vi "WebView2 Viewer.vi"(2 "ProjectRef":refnum<vi>, 4 "Extra Scripts":string, 5 "FileDependency In":map{path, T1}(c390), 6 "Options":string, 7 "OpenWebBrowser(False)":bool, 8 "error in":errorcluster, 9 "Embedd VISJS Librarya in HTMl File(False)":bool, 10 "HTMLFilePath":path, 11 "LibraryDependency":map{path, T3}(c390)) -> (0 "error out":errorcluster, 3 "HTMLFileContent":string)   [LabVIEW 2020, in "WebView2-Viewer.lvlib"] (continued)
if(this.selected=g,void 0!==this.imageObjAlt&&t){var A=this.imageObj;this.imageObj=this.imageObjAlt,this.imageObjAlt=A}}},{key:\"_getImagePadding\",value:function(){var g={top:0,right:0,bottom:0,left:0};if(this.options.imagePadding){var t=this.options.imagePadding;\"object\"==yd(t)?(g.top=t.top,g.right=t.right,g.bottom=t.bottom,g.left=t.left):(g.top=t,g.right=t,g.bottom=t,g.left=t)}return g}},{key:\"_resizeImage\",value:function(){var g,t;if(!1===this.options.shapeProperties.useImageSize){var A=1,e=1;this.imageObj.width&&this.imageObj.height&&(this.imageObj.width>this.imageObj.height?A=this.imageObj.width/this.imageObj.height:e=this.imageObj.height/this.imageObj.width),g=2*this.options.size*A,t=2*this.options.size*e}else{var C=this._getImagePadding();g=this.imageObj.width+C.left+C.right,t=this.imageObj.height+C.top+C.bottom}this.width=g,this.height=t,this.radius=.5*this.width}},{key:\"_drawRawCircle\",value:function(g,t,A,e){this.initContextForDraw(g,e),Le(g,t,A,e.size),this.performFill(g,e)}},{key:\"_drawImageAtPosition\",value:function(g,t){if(0!=this.imageObj.width){g.globalAlpha=void 0!==t.opacity?t.opacity:1,this.enableShadow(g,t);var A=1;!0===this.options.shapeProperties.interpolation&&(A=this.imageObj.width/this.width/this.body.view.scale);var e=this._getImagePadding(),C=this.left+e.left,I=this.top+e.top,i=this.width-e.left-e.right,o=this.height-e.top-e.bottom;this.imageObj.drawImageAtPosition(g,A,C,I,i,o),this.disableShadow(g,t)}}},{key:\"_drawImageLabel\",value:function(g,t,A,e,C){var I=0;if(void 0!==this.height){I=.5*this.height;var i=this.labelModule.getTextSize(g,e,C);i.lineCount>=1&&(I+=i.height/2)}var o=A+I;this.options.label&&(this.labelOffset=I),this.labelModule.draw(g,t,o,e,C,\"hanging\")}}]),A}($D);function CN(g){var t=function(){if(\"undefined\"==typeof Reflect||!MT)return!1;if(MT.sham)return!1;if(\"function\"==typeof Proxy)return!0;try{return Boolean.prototype.valueOf.call(MT(Boolean,[],(function(){}))),!0}catch(g){return!1}}();return function(){var A,e=nb(g);if(t){var C=nb(this).constructor;A=MT(e,arguments,C)}else A=e.apply(this,arguments);return Ib(this,A)}}var IN=function(g){Cb(A,g);var t=CN(A);function A(g,e,C){var I;return cn(this,A),(I=t.call(this,g,e,C))._setMargins(C),I}return kd(A,[{key:\"resize\",value:function(g){var t=arguments.length>1&&void 0!==arguments[1]?arguments[1]:this.selected,A=arguments.length>2&&void 0!==arguments[2]?arguments[2]:this.hover;if(this.needsRefresh(t,A)){var e=this.getDimensionsFromLabel(g,t,A),C=Math.max(e.width+this.margin.right+this.margin.left,e.height+this.margin.top+this.margin.bottom);this.options.size=C/2,this.width=C,this.height=C,this.radius=this.width/2}}},{key:\"draw\",value:function(g,t,A,e,C,I){this.resize(g,e,C),this.left=t-this.width/2,this.top=A-this.height/2,this._drawRawCircle(g,t,A,I),this.updateBoundingBox(t,A),this.labelModule.draw(g,this.left+this.textSize.width/2+this.margin.left,A,e,C)}},{key:\"updateBoundingBox\",value:function(g,t){this.boundingBox.top=t-this.options.size,this.boundingBox.left=g-this.options.size,this.boundingBox.right=g+this.options.size,this.boundingBox.bottom=t+this.options.size}},{key:\"distanceToBorder\",value:function(g){return g&&this.resize(g),.5*this.width}}]),A}(eN);function iN(g){var t=function(){if(\"undefined\"==typeof Reflect||!MT)return!1;if(MT.sham)return!1;if(\"function\"==typeof Proxy)return!0;try{return Boolean.prototype.valueOf.call(MT(Boolean,[],(function(){}))),!0}catch(g){return!1}}();return function(){var A,e=nb(g);if(t){var C=nb(this).constructor;A=MT(e,arguments,C)}else A=e.apply(this,arguments);return Ib(this,A)}}var oN=function(g){Cb(A,g);var t=iN(A);function A(g,e,C,I,i){var o;return cn(this,A),(o=t.call(this,g,e,C)).setImages(I,i),o}return kd(A,[{key:\"resize\",value:function(g){var t=arguments.length>1&&void 0!==arguments[1]?arguments[1]:this.selected,A=arguments.length>2&&void 0!==arguments[2]?arguments[2]:this.hover;if(void 0===this.imageObj.src||void 0===this.imageObj.width||void 0===this.imageObj.height){var e=2*this.options.size;return this.width=e,this.height=e,void(this.radius=.5*this.width)}this.needsRefresh(t,A)&&this._resizeImage()}},{key:\"draw\",value:function(g,t,A,e,C,I){this.switchImages(e),this.resize();var i=t,o=A;\"top-left\"===this.options.shapeProperties.coordinateOrigin?(this.left=t,this.top=A,i+=this.width/2,o+=this.height/2):(this.left=t-this.width/2,this.top=A-this.height/2),this._drawRawCircle(g,i,o,I),g.save(),g.clip(),this._drawImageAtPosition(g,I),g.restore(),this._drawImageLabel(g,i,o,e,C),this.updateBoundingBox(t,A)}},{key:\"updateBoundingBox\",value:function(g,t){\"top-left\"===this.options.shapeProperties.coordinateOrigin?(this.boundingBox.top=t,this.boundingBox.left=g,this.boundingBox.right=g+2*this.options.size,this.boundingBox.bottom=t+2*this.options.size):(this.boundingBox.top=t-this.options.size,this.boundingBox.left=g-this.options.size,this.boundingBox.right=g+this.options.size,this.boundingBox.bottom=t+this.options.size),this.boundingBox.left=Math.min(this.boundingBox.left,this.labelModule.size.left),this.boundingBox.right=Math.max(this.boundingBox.right,this.labelModule.size.left+this.labelModule.size.width),this.boundingBox.bottom=Math.max(this.boundingBox.bottom,this.boundingBox.bottom+this.labelOffset)}},{key:\"distanceToBorder\",value:function(g){return g&&this.resize(g),.5*this.width}}]),A}(eN);function nN(g){var t=function(){if(\"undefined\"==typeof Reflect||!MT)return!1;if(MT.sham)return!1;if(\"function\"==typeof Proxy)return!0;try{return Boolean.prototype.valueOf.call(MT(Boolean,[],(function(){}))),!0}catch(g){return!1}}();return function(){var A,e=nb(g);if(t){var C=nb(this).constructor;A=MT(e,arguments,C)}else A=e.apply(this,arguments);return Ib(this,A)}}var rN=function(g){Cb(A,g);var t=nN(A);function A(g,e,C){return cn(this,A),t.call(this,g,e,C)}return kd(A,[{key:\"resize\",value:function(g){var t=arguments.length>1&&void 0!==arguments[1]?arguments[1]:this.selected,A=arguments.length>2&&void 0!==arguments[2]?arguments[2]:this.hover,e=arguments.length>3&&void 0!==arguments[3]?arguments[3]:{size:this.options.size};if(this.needsRefresh(t,A)){var C,I;this.labelModule.getTextSize(g,t,A);var i=2*e.size;this.width=null!==(C=this.customSizeWidth)&&void 0!==C?C:i,this.height=null!==(I=this.customSizeHeight)&&void 0!==I?I:i,this.radius=.5*this.width}}},{key:\"_drawShape\",value:function(g,t,A,e,C,I,i,o){var n,r=this;return this.resize(g,I,i,o),this.left=e-this.width/2,this.top=C-this.height/2,this.initContextForDraw(g,o),(n=t,Object.prototype.hasOwnProperty.call(Ue,n)?Ue[n]:function(g){for(var t=arguments.length,A=new Array(t>1?t-1:0),e=1;e<t;e++)A[e-1]=arguments[e];CanvasRenderingContext2D.prototype[n].call(g,A)})(g,e,C,o.size),this.performFill(g,o),void 0!==this.options.icon&&void 0!==this.options.icon.code&&(g.font=(I?\"bold \":\"\")+this.height/2+\"px \"+(this.options.icon.face||\"FontAwesome\"),g.fillStyle=this.options.icon.color||\"black\",g.textAlign=\"center\",g.textBaseline=\"middle\",g.fillText(this.options.icon.code,e,C)),{drawExternalLabel:function(){if(void 0!==r.options.label){r.labelModule.calculateLabelSize(g,I,i,e,C,\"hanging\");var t=C+.5*r.height+.5*r.labelModule.size.height;r.labelModule.draw(g,e,t,I,i,\"hanging\")}r.updateBoundingBox(e,C)}}}},{key:\"updateBoundingBox\",value:function(g,t){this.boundingBox.top=t-this.options.size,this.boundingBox.left=g-this.options.size,this.boundingBox.right=g+this.options.size,this.boundingBox.bottom=t+this.options.size,void 0!==this.options.label&&this.labelModule.size.width>0&&(this.boundingBox.left=Math.min(this.boundingBox.left,this.labelModule.size.left),this.boundingBox.right=Math.max(this.boundingBox.right,this.labelModule.size.left+this.labelModule.size.width),this.boundingBox.bottom=Math.max(this.boundingBox.bottom,this.boundingBox.bottom+this.labelModule.size.height))}}]),A}($D);function sN(g,t){var A=Lh(g);if(BT){var e=BT(g);t&&(e=pc(e).call(e,(function(t){return WT(g,t).enumerable}))),A.push.apply(A,e)}return A}function aN(g){for(var t=1;t<arguments.length;t++){var A,e,C=null!=arguments[t]?arguments[t]:{};t%2?Cl(A=sN(Object(C),!0)).call(A,(function(t){rb(g,t,C[t])})):HT?AD(g,HT(C)):Cl(e=sN(Object(C))).call(e,(function(t){fT(g,t,WT(C,t))}))}return g}function dN(g){var t=function(){if(\"undefined\"==typeof Reflect||!MT)return!1;if(MT.sham)return!1;if(\"function\"==typeof Proxy)return!0;try{return Boolean.prototype.valueOf.call(MT(Boolean,[],(function(){}))),!0}catch(g){return!1}}();return function(){var A,e=nb(g);if(t){var C=nb(this).constructor;A=MT(e,arguments,C)}else A=e.apply(this,arguments);return Ib(this,A)}}var hN=function(g){Cb(A,g);var t=dN(A);function A(g,e,C,I){var i;return cn(this,A),(i=t.call(this,g,e,C,I)).ctxRenderer=I,i}return kd(A,[{key:\"draw\",value:function(g,t,A,e,C,I){this.resize(g,e,C,I),this.left=t-this.width/2,this.top=A-this.height/2,g.save();var i=this.ctxRenderer({ctx:g,id:this.options.id,x:t,y:A,state:{selected:e,hover:C},style:aN({},I),label:this.options.label});if(null!=i.drawNode&&i.drawNode(),g.restore(),i.drawExternalLabel){var o=i.drawExternalLabel;i.drawExternalLabel=function(){g.save(),o(),g.restore()}}return i.nodeDimensions&&(this.customSizeWidth=i.nodeDimensions.width,this.customSizeHeight=i.nodeDimensions.height),i}},{key:\"distanceToBorder\",value:function(g,t){return this._distanceToBorder(g,t)}}]),A}(rN);function lN(g){var t=function(){if(\"undefined\"==typeof Reflect||!MT)return!1;if(MT.sham)return!1;if(\"function\"==typeof Proxy)return!0;try{return Boolean.prototype.valueOf.call(MT(Boolean,[],(function(){}))),!0}catch(g){return!1}}();return function(){var A,e=nb(g);if(t){var C=nb(this).constructor;A=MT(e,arguments,C)}else A=e.apply(this,arguments);return Ib(this,A)}}var cN=function(g){Cb(A,g);var t=lN(A);function A(g,e,C){var I;return cn(this,A),(I=t.call(this,g,e,C))._setMargins(C),I}return kd(A,[{key:\"resize\",value:function(g,t,A){if(this.needsRefresh(t,A)){var e=this.getDimensionsFromLabel(g,t,A).width+this.margin.right+this.margin.left;this.width=e,this.height=e,this.radius=this.width/2}}},{key:\"draw\",value:function(g,t,A,e,C,I){this.resize(g,e,C),this.left=t-this.width/2,this.top=A-this.height/2,this.initContextForDraw(g,I),We(g,t-this.width/2,A-this.height/2,this.width,this.height),this.performFill(g,I),this.updateBoundingBox(t,A,g,e,C),this.labelModule.draw(g,this.left+this.textSize.width/2+this.margin.left,this.top+this.textSize.height/2+this.margin.top,e,C)}},{key:\"distanceToBorder\",value:function(g,t){return this._distanceToBorder(g,t)}}]),A}($D);function uN(g){var t=function(){if(\"undefined\"==typeof Reflect||!MT)return!1;if(MT.sham)return!1;if(\"function\"==typeof Proxy)return!0;try{return Boolean.prototype.valueOf.call(MT(Boolean,[],(function(){}))),!0}catch(g){return!1}}();return function(){var A,e=nb(g);if(t){var C=nb(this).constructor;A=MT(e,arguments,C)}else A=e.apply(this,arguments);return Ib(this,A)}}var pN=function(g){Cb(A,g);var t=uN(A);function A(g,e,C){return cn(this,A),t.call(this,g,e,C)}return kd(A,[{key:\"draw\",value:function(g,t,A,e,C,I){return this._drawShape(g,\"diamond\",4,t,A,e,C,I)}},{key:\"distanceToBorder\",value:function(g,t){return this._distanceToBorder(g,t)}}]),A}(rN);function fN(g){var t=function(){if(\"undefined\"==typeof Reflect||!MT)return!1;if(MT.sham)return!1;if(\"function\"==typeof Proxy)return!0;try{return Boolean.prototype.valueOf.call(MT(Boolean,[],(function(){}))),!0}catch(g){return!1}}();return function(){var A,e=nb(g);if(t){var C=nb(this).constructor;A=MT(e,arguments,C)}else A=e.apply(this,arguments);return Ib(this,A)}}var vN=function(g){Cb(A,g);var t=fN(A);function A(g,e,C){return cn(this,A),t.call(this,g,e,C)}return kd(A,[{key:\"draw\",value:function(g,t,A,e,C,I){return this._drawShape(g,\"circle\",2,t,A,e,C,I)}},{key:\"distanceToBorder\",value:function(g){return g&&this.resize(g),this.options.size}}]),A}(rN);function yN(g){var t=function(){if(\"undefined\"==typeof Reflect||!MT)return!1;if(MT.sham)return!1;if(\"function\"==typeof Proxy)return!0;try{return Boolean.prototype.valueOf.call(MT(Boolean,[],(function(){}))),!0}catch(g){return!1}}();return function(){var A,e=nb(g);if(t){var C=nb(this).constructor;A=MT(e,arguments,C)}else A=e.apply(this,arguments);return Ib(this,A)}}var mN=function(g){Cb(A,g);var t=yN(A);function A(g,e,C){return cn(this,A),t.call(this,g,e,C)}return kd(A,[{key:\"resize\",value:function(g){var t=arguments.length>1&&void 0!==arguments[1]?arguments[1]:this.selected,A=arguments.length>2&&void 0!==arguments[2]?arguments[2]:this.hover;if(this.needsRefresh(t,A)){var e=this.getDimensionsFromLabel(g,t,A);this.height=2*e.height,this.width=e.width+e.height,this.radius=.5*this.width}}},{key:\"draw\",value:function(g,t,A,e,C,I){this.resize(g,e,C),this.left=t-.5*this.width,this.top=A-.5*this.height,this.initContextForDraw(g,I),Ye(g,this.left,this.top,this.width,this.height),this.performFill(g,I),this.updateBoundingBox(t,A,g,e,C),this.labelModule.draw(g,t,A,e,C)}},{key:\"distanceToBorder\",value:function(g,t){g&&this.resize(g);var A=.5*this.width,e=.5*this.height,C=Math.sin(t)*A,I=Math.cos(t)*e;return A*e/Math.sqrt(C*C+I*I)}}]),A}($D);function bN(g){var t=function(){if(\"undefined\"==typeof Reflect||!MT)return!1;if(MT.sham)return!1;if(\"function\"==typeof Proxy)return!0;try{return Boolean.prototype.valueOf.call(MT(Boolean,[],(function(){}))),!0}catch(g){return!1}}();return function(){var A,e=nb(g);if(t){var C=nb(this).constructor;A=MT(e,arguments,C)}else A=e.apply(this,arguments);return Ib(this,A)}}var wN=function(g){Cb(A,g);var t=bN(A);function A(g,e,C){var I;return cn(this,A),(I=t.call(this,g,e,C))._setMargins(C),I}return kd(A,[{key:\"resize\",value:function(g,t,A){this.needsRefresh(t,A)&&(this.iconSize={width:Number(this.options.icon.size),height:Number(this.options.icon.size)},this.width=this.iconSize.width+this.margin.right+this.margin.left,this.height=this.iconSize.height+this.margin.top+this.margin.bottom,this.radius=.5*this.width)}},{key:\"draw\",value:function(g,t,A,e,C,I){var i=this;return this.resize(g,e,C),this.options.icon.size=this.options.icon.size||50,this.left=t-this.width/2,this.top=A-this.height/2,this._icon(g,t,A,e,C,I),{drawExternalLabel:function(){if(void 0!==i.options.label){i.labelModule.draw(g,i.left+i.iconSize.width/2+i.margin.left,A+i.height/2+5,e)}i.updateBoundingBox(t,A)}}}},{key:\"updateBoundingBox\",value:function(g,t){if(this.boundingBox.top=t-.5*this.options.icon.size,this.boundingBox.left=g-.5*this.options.icon.size,this.boundingBox.right=g+.5*this.options.icon.size,this.boundingBox.bottom=t+.5*this.options.icon.size,void 0!==this.options.label&&this.labelModule.size.width>0){this.boundingBox.left=Math.min(this.boundingBox.left,this.labelModule.size.left),this.boundingBox.right=Math.max(this.boundingBox.right,this.labelModule.size.left+this.labelModule.size.width),this.boundingBox.bottom=Math.max(this.boundingBox.bottom,this.boundingBox.bottom+this.labelModule.size.height+5)}}},{key:\"_icon\",value:function(g,t,A,e,C,I){var i=Number(this.options.icon.size);void 0!==this.options.icon.code?(g.font=[null!=this.options.icon.weight?this.options.icon.weight:e?\"bold\":\"\",(null!=this.options.icon.weight&&e?5:0)+i+\"px\",this.options.icon.face].join(\" \"),g.fillStyle=this.options.icon.color||\"black\",g.textAlign=\"center\",g.textBaseline=\"middle\",this.enableShadow(g,I),g.fillText(this.options.icon.code,t,A),this.disableShadow(g,I)):console.error(\"When using the icon shape, you need to define the code in the icon options object. This can be done per node or globally.\")}},{key:\"distanceToBorder\",value:function(g,t){return this._distanceToBorder(g,t)}}]),A}($D);function kN(g){var t=function(){if(\"undefined\"==typeof Reflect||!MT)return!1;if(MT.sham)return!1;if(\"function\"==typeof Proxy)return!0;try{return Boolean.prototype.valueOf.call(MT(Boolean,[],(function(){}))),!0}catch(g){return!1}}();return function(){var A,e=nb(g);if(t){var C=nb(this).constructor;A=MT(e,arguments,C)}else A=e.apply(this,arguments);return Ib(this,A)}}var xN=function(g){Cb(A,g);var t=kN(A);function A(g,e,C,I,i){var o;return cn(this,A),(o=t.call(this,g,e,C)).setImages(I,i),o}return kd(A,[{key:\"resize\",value:function(g){var t=arguments.length>1&&void 0!==arguments[1]?arguments[1]:this.selected,A=arguments.length>2&&void 0!==arguments[2]?arguments[2]:this.hover;if(void 0===this.imageObj.src||void 0===this.imageObj.width||void 0===this.imageObj.height){var e=2*this.options.size;return this.width=e,void(this.height=e)}this.needsRefresh(t,A)&&this._resizeImage()}},{key:\"draw\",value:function(g,t,A,e,C,I){g.save(),this.switchImages(e),this.resize();var i=t,o=A;if(\"top-left\"===this.options.shapeProperties.coordinateOrigin?(this.left=t,this.top=A,i+=this.width/2,o+=this.height/2):(this.left=t-this.width/2,this.top=A-this.height/2),!0===this.options.shapeProperties.useBorderWithImage){var n=this.options.borderWidth,r=this.options.borderWidthSelected||2*this.options.borderWidth,s=(e?r:n)/this.body.view.scale;g.lineWidth=Math.min(this.width,s),g.beginPath();var a=e?this.options.color.highlight.border:C?this.options.color.hover.border:this.options.color.border,d=e?this.options.color.highlight.background:C?this.options.color.hover.background:this.options.color.background;void 0!==I.opacity&&(a=ev(a,I.opacity),d=ev(d,I.opacity)),g.strokeStyle=a,g.fillStyle=d,g.rect(this.left-.5*g.lineWidth,this.top-.5*g.lineWidth,this.width+g.lineWidth,this.height+g.lineWidth),Bu(g).call(g),this.performStroke(g,I),g.closePath()}this._drawImageAtPosition(g,I),this._drawImageLabel(g,i,o,e,C),this.updateBoundingBox(t,A),g.restore()}},{key:\"updateBoundingBox\",value:function(g,t){this.resize(),\"top-left\"===this.options.shapeProperties.coordinateOrigin?(this.left=g,this.top=t):(this.left=g-this.width/2,this.top=t-this.height/2),this.boundingBox.left=this.left,this.boundingBox.top=this.top,this.boundingBox.bottom=this.top+this.height,this.boundingBox.right=this.left+this.width,void 0!==this.options.label&&this.labelModule.size.width>0&&(this.boundingBox.left=Math.min(this.boundingBox.left,this.labelModule.size.left),this.boundingBox.right=Math.max(this.boundingBox.right,this.labelModule.size.left+this.labelModule.size.width),this.boundingBox.bottom=Math.max(this.boundingBox.bottom,this.boundingBox.bottom+this.labelOffset))}},{key:\"distanceToBorder\",value:function(g,t){return this._distanceToBorder(g,t)}}]),A}(eN);function EN(g){var t=function(){if(\"undefined\"==typeof Reflect||!MT)return!1;if(MT.sham)return!1;if(\"function\"==typeof Proxy)return!0;try{return Boolean.prototype.valueOf.call(MT(Boolean,[],(function(){}))),!0}catch(g){return!1}}();return function(){var A,e=nb(g);if(t){var C=nb(this).constructor;A=MT(e,arguments,C)}else A=e.apply(this,arguments);return Ib(this,A)}}var ON=function(g){Cb(A,g);var t=EN(A);function A(g,e,C){return cn(this,A),t.call(this,g,e,C)}return kd(A,[{key:\"draw\",value:function(g,t,A,e,C,I){return this._drawShape(g,\"square\",2,t,A,e,C,I)}},{key:\"distanceToBorder\",value:function(g,t){return this._distanceToBorder(g,t)}}]),A}(rN);function TN(g){var t=function(){if(\"undefined\"==typeof Reflect||!MT)return!1;if(MT.sham)return!1;if(\"function\"==typeof Proxy)return!0;try{return Boolean.prototype.valueOf.call(MT(Boolean,[],(function(){}))),!0}catch(g){return!1}}();return function(){var A,e=nb(g);if(t){var C=nb(this).constructor;A=MT(e,arguments,C)}else A=e.apply(this,arguments);return Ib(this,A)}}var DN=function(g){Cb(A,g);var t=TN(A);function A(g,e,C){return cn(this,A),t.call(this,g,e,C)}return kd(A,[{key:\"draw\",value:function(g,t,A,e,C,I){return this._drawShape(g,\"hexagon\",4,t,A,e,C,I)}},{key:\"distanceToBorder\",value:function(g,t){return this._distanceToBorder(g,t)}}]),A}(rN);function NN(g){var t=function(){if(\"undefined\"==typeof Reflect||!MT)return!1;if(MT.sham)return!1;if(\"function\"==typeof Proxy)return!0;try{return Boolean.prototype.valueOf.call(MT(Boolean,[],(function(){}))),!0}catch(g){return!1}}();return function(){var 
